vi "multi-graph-example-events.vi"() -> ()   [LabVIEW 2017]
panel:
  out "cycle #":i32
  in  "LSI-U CH labels":string[](array[string])
  out "labels S1":string[](array[string])
  in  "GraphU2 SEL":i32[](array[numeric])
  in  "log/linear":bool
  in  "stop":bool
  out "Graph1 (4-10K)":cluster{timestamp[], dbl[]}[](graph)
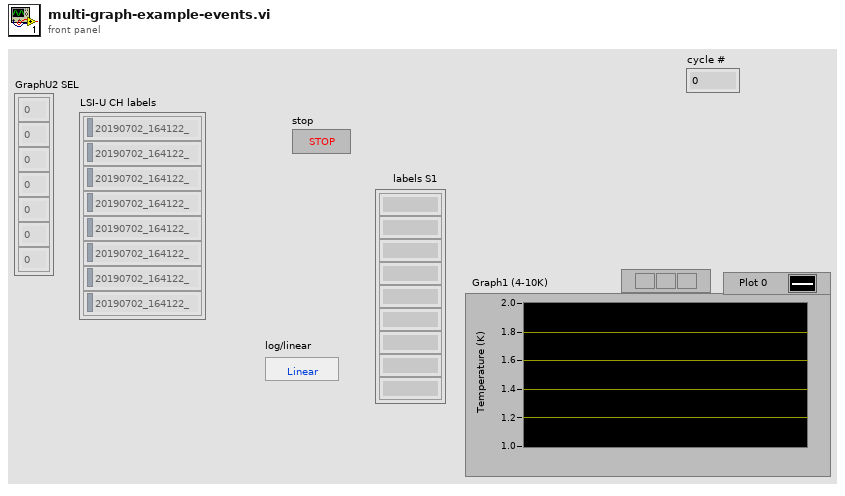
[diagram p1: front panel]
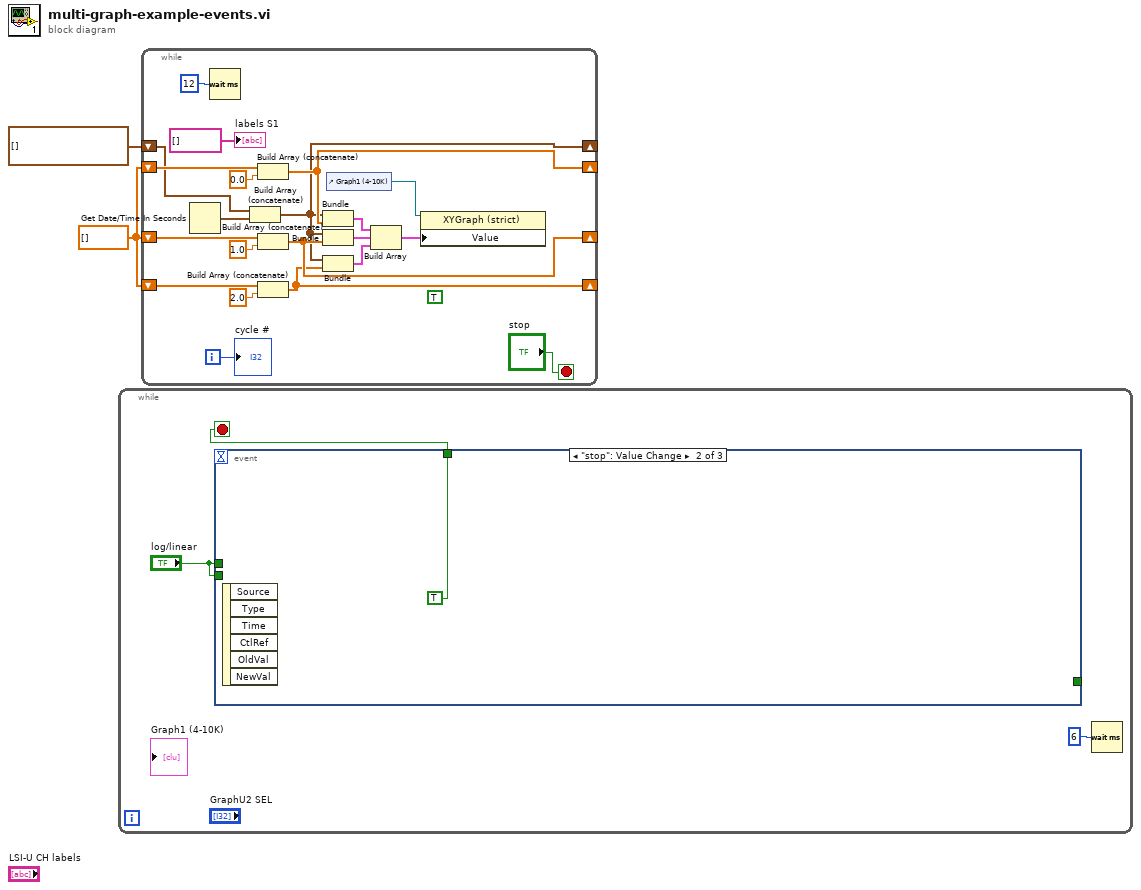
[diagram p0: block diagram]
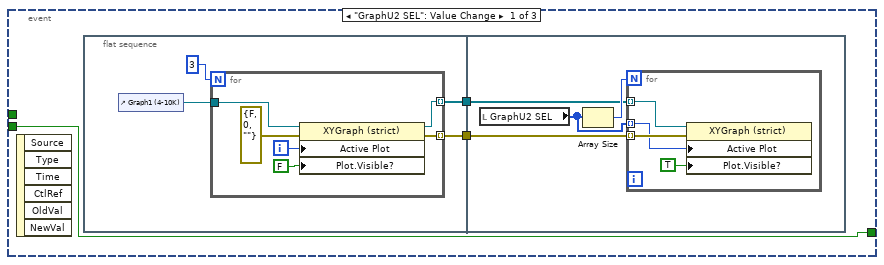
[diagram p2: hidden frame]
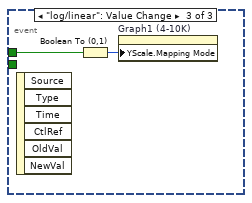
[diagram p3: hidden frame]
diagram:
  w1 = dbl[] []
  n1 = while {
    stop <- w3 stop-if-true
    n2 = event shown="[1] \"stop\": Value Change" {
      selector: _ -> [_ _ _]
      dyn-events: _ -> [_ _ _]
      timeout: _ -> [_ _ _]
      tunnel: "log/linear" -> [w8 _ _]
      tunnel: [w8 _ _] -> _
      tunnel: "log/linear" -> [_ _ w28]
      tunnel: [_ TRUE _] -> w3
      event "GraphU2 SEL": Value Change {
        n3 = event-data() -> ()  [unwired: 1 in, 6 out]
        n4 = flat-sequence {
          tunnel: [w10] -> w7
          tunnel: [w9] -> w6
          tunnel: w7 -> [w20]
          tunnel: w6 -> [w19]
          frame #0 {
            n5 = control-ref of="Graph1 (4-10K)"() -> (w11:refnum<vi>)
            n6 = for {
              N: 3 -> [_]
              tunnel: w11 -> [w18]
              tunnel: [w14] -> w10 mode=indexing
              tunnel: [w13] -> w9 mode=indexing
              i -> [w16]
              n7 = property class="XYGraph (strict)"(reference=w18, error in=errorcluster {"status"=FALSE, "code"=0, "source"=""} ("error in (no error)"), "Active Plot"=w16, "Plot.Visible?"=FALSE ("Plot.Visible")) -> (reference out=w14:refnum<vi>, error out=w13:errorcluster)
            }
          }
          frame #1 {
            n8 = local read "GraphU2 SEL"() -> (w21:i32[])
            n9 = Array Size(array=w21) -> (size(s)=w22:i32)
            n10 = for {
              N: w22 -> [_]
              tunnel: w21 -> [w24] mode=indexing
              tunnel: w20 -> [w26] mode=indexing
              tunnel: w19 -> [w25] mode=indexing
              n11 = property class="XYGraph (strict)"(reference=w26, error in=w25, "Active Plot"=w24, "Plot.Visible?"=TRUE ("Plot.Visible")) -> ()  [unwired: 2 out]
            }
          }
        }
      }
      event "stop": Value Change {
        n12 = event-data() -> ()  [unwired: 1 in, 6 out]
      }
      event "log/linear": Value Change {
        n13 = event-data() -> ()  [unwired: 1 in, 6 out]
        n14 = Boolean To (0,1)(Boolean=w28) -> (0, 1=w29:i16)
        n15 = property on="Graph1 (4-10K)" class="XYGraph (strict)"("YScale.Mapping Mode"=w29) -> ()  [unwired: 2 in, 2 out]
      }
    }
    n16 = Wait (ms)(milliseconds to wait=u32 6) -> ()  [unwired: 1 out]
  }
  n17 = while {
    shift-right: [w44] -> _
    shift-left: w1 -> [w49]
    shift-right: [w38] -> _
    shift-left: timestamp[] [] -> [w47]
    shift-right: [w41] -> _
    shift-left: w1 -> [w42]
    shift-right: [w37] -> _
    shift-left: w1 -> [w39]
    i -> [w32]
    stop <- "stop" stop-if-true
    (unwired) TRUE ("Visible")
    n18 = Get Date/Time In Seconds() -> (seconds since 1Jan1904=w48:timestamp)
    n19 = Wait (ms)(milliseconds to wait=u32 12) -> ()  [unwired: 1 out]
    n20 = Build Array (concatenate)(w47, w48) -> (w38:timestamp[])
    n21 = Build Array (concatenate)(w49, 0.0) -> (w44:dbl[])
    n22 = Build Array (concatenate)(w42, 1.0) -> (w41:dbl[])
    n23 = Build Array (concatenate)(w39, 2.0) -> (w37:dbl[])
    n24 = Bundle(w38, w44) -> (w36:cluster{timestamp[], dbl[]})  [unwired: 1 in]
    n25 = Bundle(w38, w41) -> (w35:cluster{timestamp[], dbl[]})  [unwired: 1 in]
    n26 = Bundle(w38, w37) -> (w34:cluster{timestamp[], dbl[]})  [unwired: 1 in]
    n27 = control-ref of="Graph1 (4-10K)"() -> (w31:refnum<vi>)
    n28 = Build Array(w36, w35, w34) -> (w30:cluster{timestamp[], dbl[]}[])
    n29 = property class="XYGraph (strict)"(reference=w31, "Value"=w30) -> ()  [unwired: 1 in, 2 out]
    "labels S1" <- string[] []
    "cycle #" <- w32
  }
